vi "Configure.vi"(8 "error in (no error)":errorcluster, 10 "Parameters":variant, 11 "Assembler in":refnum<class "Assembler.lvclass">) -> (0 "error out":errorcluster, 3 "Assembler out":refnum<class "Assembler.lvclass">)   [LabVIEW 2019, in "TimingDRV Engine.lvlib" / "Assembler.lvclass"]
uses:
  Assembler.lvclass
  C:/Users/XEnderMD/Desktop/CD Project Tools/Source/Engine/Parent Classes/Process/Process.lvclass
  TypeDefs/Assembler Configuration.ctl
  TypeDefs/Process Configuration.ctl
  Parent Classes/Process/Process.lvclass
  <vilib>/NI VeriStand/Custom Device API/Custom Device Engine Event Ref.ctl
  <vilib>/NI VeriStand/Custom Device API/Message (Byte Array).ctl
  <vilib>/NI VeriStand/Custom Device API/Message Response (Byte Array).ctl
  <vilib>/NI VeriStand/Custom Device API/Message (String).ctl
  <vilib>/NI VeriStand/Custom Device API/Message Response (String).ctl
  Parent Classes/Process/Process.lvclass/Process.ctl
  Assembler.lvclass/Assembler.ctl
  <vilib>/NI VeriStand/Custom Device API/Custom Device API.lvlib
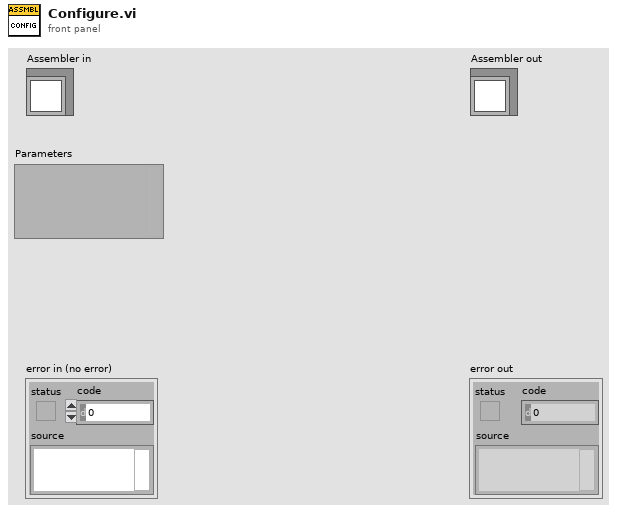
[diagram p1: front panel]
types:
  T1 = typedef "TimingDRV Engine.lvlib/Assembler.lvclass/Assembler Configuration.ctl" = cluster{"Process Settings":T2, "Processes":refnum<class "Process.lvclass">[], "CD Engine Event Ref":T3}
  T2 = typedef "TimingDRV Engine.lvlib/Assembler.lvclass/Process Configuration.ctl" = cluster{"Process Timeout":dbl}
  T3 = typedef "Custom Device API.lvlib/Custom Device Engine Event Ref.ctl" = refnum<event-registration>
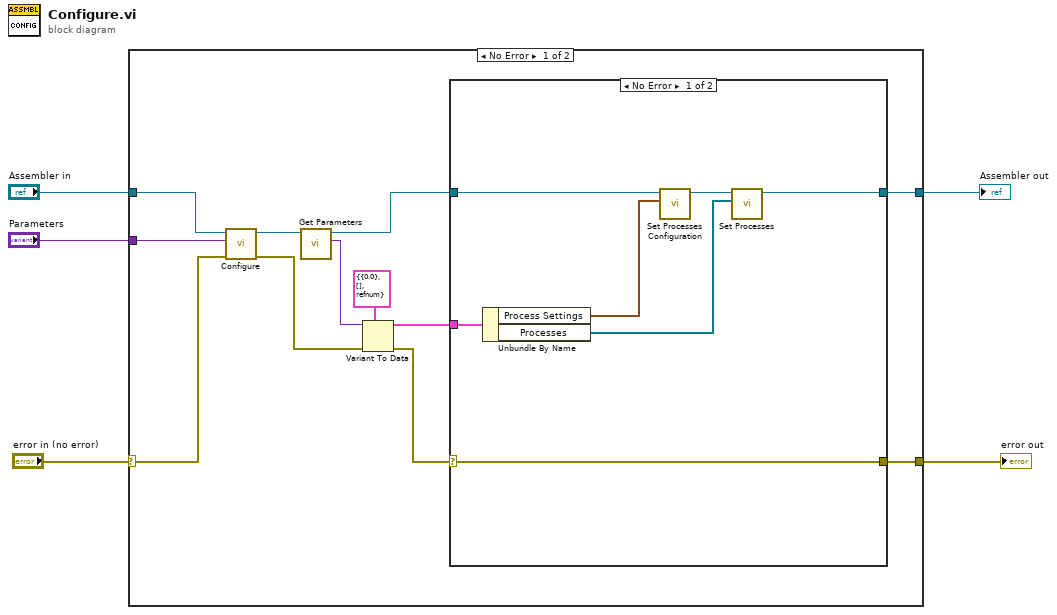
[diagram p0: block diagram]
diagram:
  n1 = case shown="No Error" "error in (no error)" {
    selector: "error in (no error)" -> [w7 w28]
    tunnel: "Parameters" -> [w17 _]
    tunnel: "Assembler in" -> [w16 w27]
    tunnel: [w10 w27] -> w3
    tunnel: [w6 w28] -> w1
    frame No Error {
      n2 = call-parent "Configure.vi"("error in (no error)"=w7, "Parameters"=w17, "Process in"=w16) -> ("error out"=w8:errorcluster, "Process out"=w13:refnum<class "Assembler.lvclass">)  [unwired: 7 in]
      n3 = call "Get Parameters.vi"("Process in"=w13) -> ("Parameters"=w15:variant, "Process out"=w11:refnum<class "Assembler.lvclass">)  [unwired: 9 in]
      n4 = Variant To Data(error in=w8, type=T1 {"Process Settings"={"Process Timeout"=0.0}, "Processes"=[], "CD Engine Event Ref"=refnum} ("Assembler Configuration"), Variant=w15) -> (data=w12:T1, error out=w9:errorcluster)
      n5 = case shown="No Error" w9 {
        selector: w9 -> [w19 w26]
        tunnel: w12 -> [w24 _]
        tunnel: w11 -> [w23 w25]
        tunnel: [w18 w25] -> w10
        tunnel: [w19 w26] -> w6
        frame No Error {
          n6 = Unbundle By Name(w24) -> ("Process Settings"=w22:T2, "Processes"=w20:refnum<class "Process.lvclass">[])
          n7 = call "Set Processes Configuration.vi"("Process Settings"=w22, "Assembler in"=w23) -> ("Assembler out"=w21:refnum<class "Assembler.lvclass">)  [unwired: 9 in]
          n8 = call "Set Processes.vi"("Processes"=w20, "Assembler in"=w21) -> ("Assembler out"=w18:refnum<class "Assembler.lvclass">)  [unwired: 9 in]
        }
        frame Error {
        }
      }
    }
    frame Error {
    }
  }
  "error out" <- w1
  "Assembler out" <- w3
